vi "Unit Test Preserve wired non-serialized data (Less-Specific) True Error.vi"() -> ()   [LabVIEW 2019, in "Sports Unit Tests.lvclass"]
uses:
  Sports Unit Tests.lvclass
  <userlib>/Blue Origin/BlueSerialization/BlueSerializer/DeserializeOptions.ctl
  <userlib>/Blue Origin/BlueSerialization/BlueSerializer/DeserializeSlicingOptions.ctl
  <userlib>/Blue Origin/BlueSerialization/BlueSerializer/DeserializeMutationOptions.ctl
  <userlib>/Blue Origin/BlueSerialization/BlueSerializer/DeserializePreservationOptions.ctl
  <userlib>/Blue Origin/BlueSerialization/BlueSerializer/PreserveNonWiredDataOption.ctl
  Classes/The Waterboy/The Waterboy.lvclass
  C:/DSCE code/Serialization/blueserializationdemo/Test/Sports/Classes/Human/Human.lvclass
  C:/DSCE code/Serialization/blueserializationdemo/Test/Sports/Classes/Sports Player/Sports Player.lvclass
  C:/DSCE code/Serialization/blueserializationdemo/Test/Sports/Classes/Golf Player/Golf Player.lvclass
  C:/DSCE code/Serialization/blueserializationdemo/Test/Sports/Classes/Adam Sandler/Adam Sandler.lvclass
  Classes/Adam Sandler/Adam Sandler.lvclass
  Classes/Human/Human.lvclass/Human.ctl
  Classes/Sports Player/Sports Player.lvclass/Sports Player.ctl
  Classes/Golf Player/Golf Player.lvclass/Golf Player.ctl
  Classes/Adam Sandler/Adam Sandler.lvclass/Adam Sandler.ctl
  Classes/Human/Write Age (years).vi
  Classes/Human/Write alive_.vi
  Classes/Human/Write Height (ft).vi
  Classes/Human/Write Name.vi
  Classes/Sports Player/Write Earnings (dollars).vi
  Classes/Sports Player/Write Professional_.vi
  Classes/Sports Player/Write Sponsor.vi
  Classes/Golf Player/Write # holes in one.vi
  Classes/Golf Player/Write League.vi
  Classes/Golf Player/Write longest drive (ft).vi
  Classes/Adam Sandler/Write Movie Name.vi
  Classes/Adam Sandler/Write Private number.vi
  Classes/Adam Sandler/Write Secret phrase.vi
  <vilib>/Utility/error.llb/Clear Errors.vi
  <vilib>/Utility/LVClass/Get LV Class Name.vi
  <vilib>/addons/_JKI Toolkits/Caraya/classes/Test/Define Test.vi
  <vilib>/addons/_JKI Toolkits/Caraya/classes/Assert/Assert.vi
  <vilib>/addons/_JKI Toolkits/Caraya/classes/Assert/Assert Error.vi
  <vilib>/addons/_JKI Toolkits/Caraya/classes/Assert/Assert Equal Value_Variant.vi
  <userlib>/Blue Origin/BlueSerialization/BlueSerializer/BlueSerializer.lvclass
panel:
  out "Table":string[][](table)
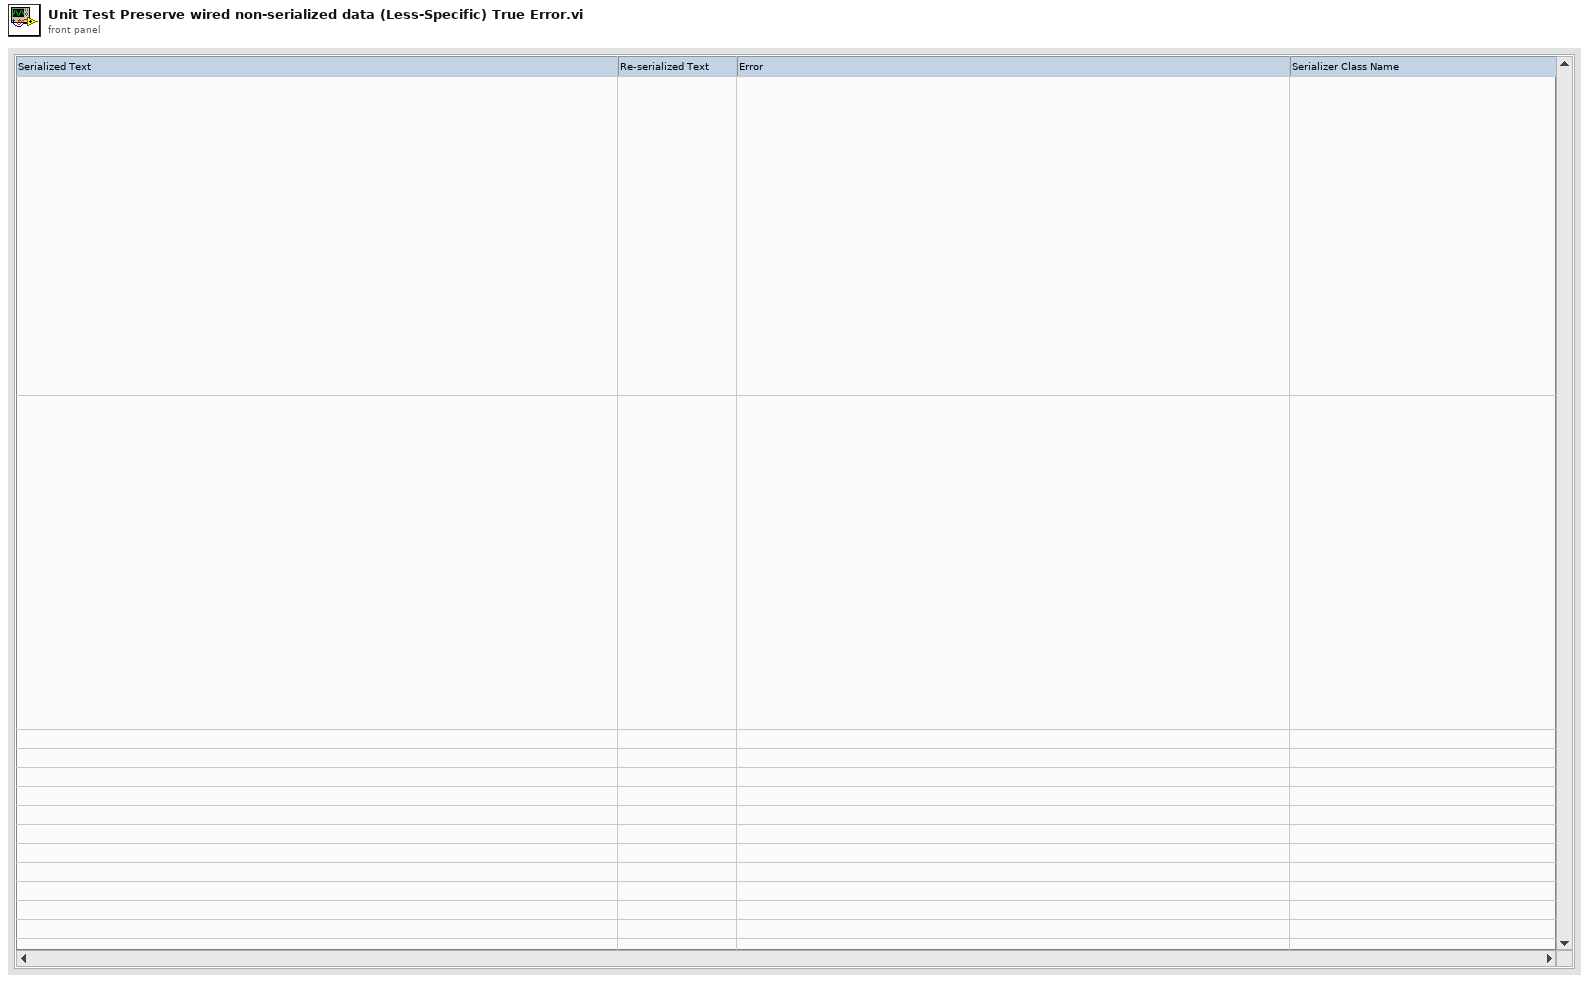
[diagram p1: front panel]
types:
  T1 = typedef "BlueSerialization.lvlib/BlueSerializer.lvclass/PreserveNonWiredDataOption.ctl" = enum16{"Don't preserve", "Preserve (error on less-specific wired types)", "Preserve (except on less-specific wired types)"}
  T2 = typedef "BlueSerialization.lvlib/BlueSerializer.lvclass/DeserializeOptions.ctl" = cluster{"deserialize non-BlueSerializable objects from hex?":bool, "expand objects on type conflict?":bool, "Slicing":T3, "Mutation Options":T4, "Preservation Options":T5}
  T3 = typedef "BlueSerialization.lvlib/BlueSerializer.lvclass/DeserializeSlicingOptions.ctl" = cluster{"slice flattened object data on error?":bool, "sliceable class names":string[]}
  T4 = typedef "BlueSerialization.lvlib/BlueSerializer.lvclass/DeserializeMutationOptions.ctl" = cluster{"error on inserted parent levels?":bool, "\terror on obsolete parent levels?":bool}
  T5 = typedef "BlueSerialization.lvlib/BlueSerializer.lvclass/DeserializePreservationOptions.ctl" = cluster{"Preserve wired serialized data?":bool, "Preserve wired non-serialized data":T1}
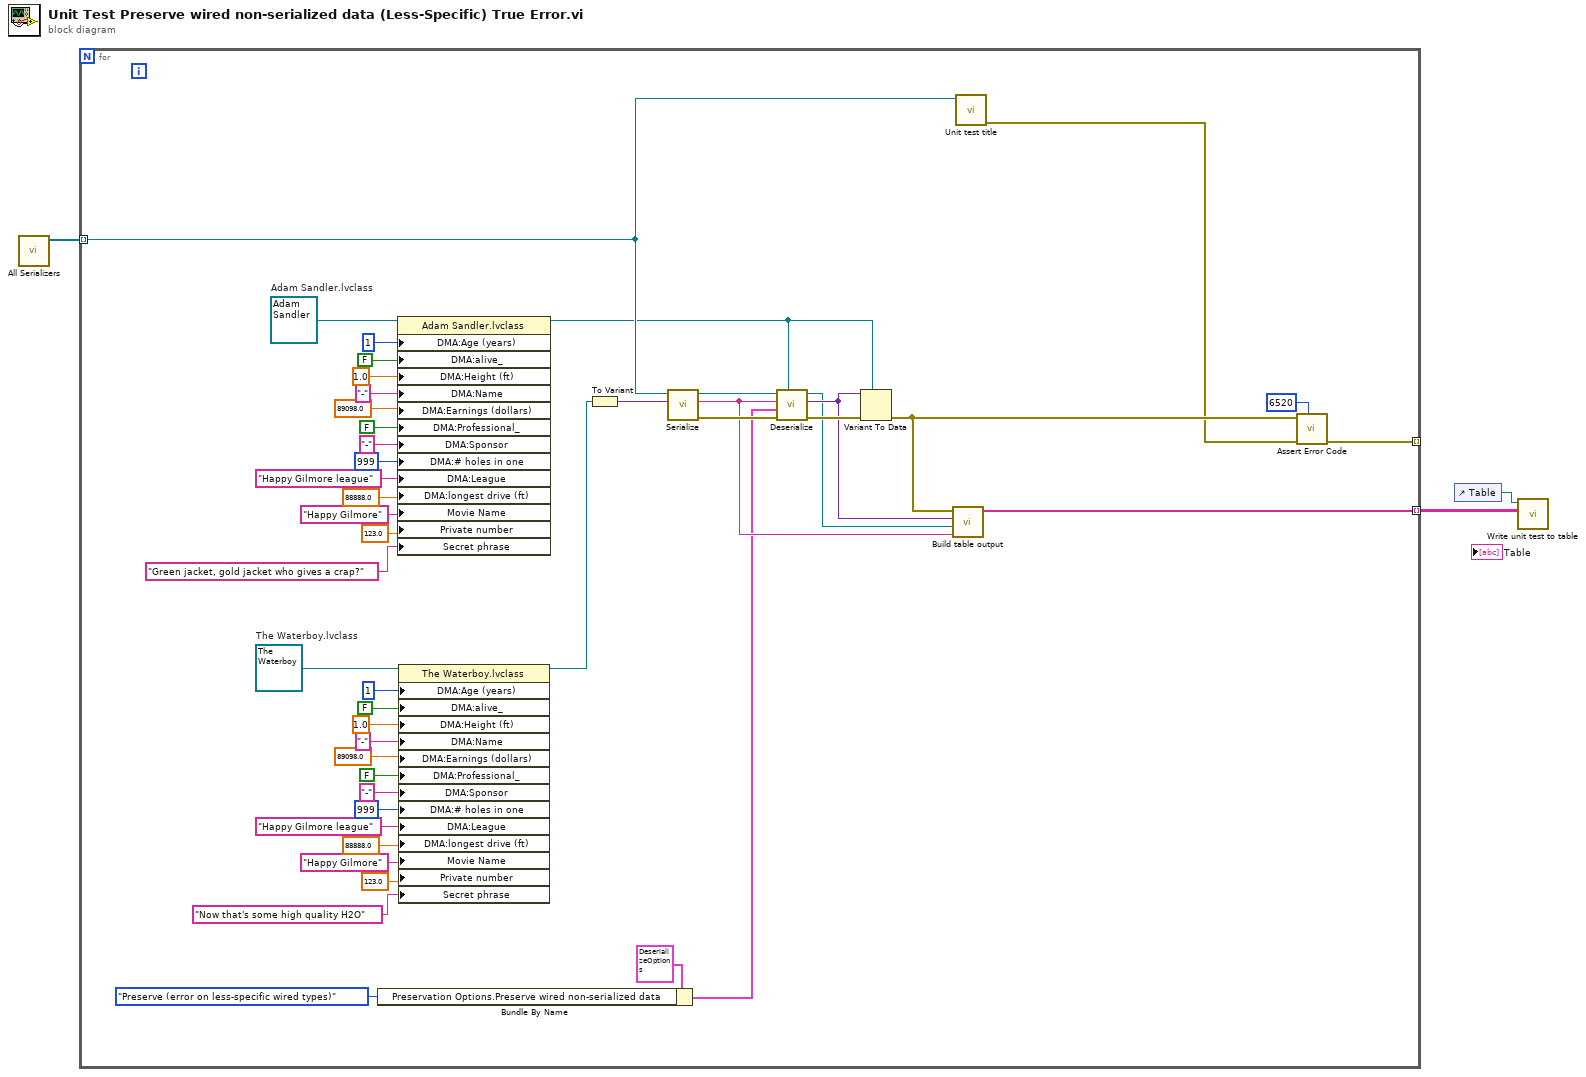
[diagram p0: block diagram]
diagram:
  n1 = call "All Serializers.vi"() -> ("All serializers"=w2:refnum<class "BlueSerializer.lvclass">[])  [unwired: 11 in]
  n2 = for {
    tunnel: w2 -> [w26] mode=indexing
    tunnel: [w5] -> _ mode=indexing
    tunnel: [w35] -> w1 mode=indexing
    w9 = refnum<class "Adam Sandler.lvclass"> refnum  # Adam Sandler.lvclass
    w10 = refnum<class "The Waterboy.lvclass"> refnum  # The Waterboy.lvclass
    n3 = Bundle By Name(cluster=T2 {"deserialize non-BlueSerializable objects from hex?"=FALSE, "expand objects on type conflict?"=FALSE, "Slicing"={"slice flattened object data on error?"=FALSE, "sliceable class names"=[]}, "Mutation Options"={"error on inserted parent levels?"=FALSE, "\terror on obsolete parent levels?"=FALSE}, "Preservation Options"={"Preserve wired serialized data?"=FALSE, "Preserve wired non-serialized data"=enum."Don't preserve"}} ("Deserialize Options"), "Preservation Options.Preserve wired non-serialized data"=PreserveNonWiredDataOption."Preserve (error on less-specific wired types)") -> (w27:T2)
    n4 = property on="Property Node" class="Adam Sandler.lvclass"(reference=w9, "DMA:Age (years)"=u16 1 ("Age (years)"), "DMA:alive_"=FALSE ("alive_"), "DMA:Height (ft)"=1.0 ("Height (ft)"), "DMA:Name"="-" ("Name"), "DMA:Earnings (dollars)"=89098.0 ("Earnings (dollars)"), "DMA:Professional_"=FALSE ("Professional_"), "DMA:Sponsor"="-" ("Sponsor"), "DMA:# holes in one"=999 ("# holes in one"), "DMA:League"="Happy Gilmore league" ("League"), "DMA:longest drive (ft)"=88888.0 ("longest drive (ft)"), "Movie Name"="Happy Gilmore", "Private number"=123.0, "Secret phrase"="Green jacket, gold jacket who gives a crap?") -> (reference out=w11:refnum<class "Adam Sandler.lvclass">)  [unwired: 1 in, 1 out]
    n5 = property on="Property Node" class="The Waterboy.lvclass"(reference=w10, "DMA:Age (years)"=u16 1 ("Age (years)"), "DMA:alive_"=FALSE ("alive_"), "DMA:Height (ft)"=1.0 ("Height (ft)"), "DMA:Name"="-" ("Name"), "DMA:Earnings (dollars)"=89098.0 ("Earnings (dollars)"), "DMA:Professional_"=FALSE ("Professional_"), "DMA:Sponsor"="-" ("Sponsor"), "DMA:# holes in one"=999 ("# holes in one"), "DMA:League"="Happy Gilmore league" ("League"), "DMA:longest drive (ft)"=88888.0 ("longest drive (ft)"), "Movie Name"="Happy Gilmore", "Private number"=123.0, "Secret phrase"="Now that's some high quality H2O") -> (reference out=w12:refnum<class "The Waterboy.lvclass">)  [unwired: 1 in, 1 out]
    n6 = To Variant(anything=w12) -> (Variant=w47:variant)
    n7 = call <userlib>:"Serialize.vi"("Anything"=w47, "BlueSerializer in"=w26) -> ("error out"=w49:errorcluster, "Serialized Text"=w36:string, "BlueSerializer out"=w48:refnum<class "BlueSerializer.lvclass">)  [unwired: 7 in]
    n8 = call <userlib>:"Deserialize.vi"("Anything"=w11, "error in (no error)"=w49, "Deserialize Options"=w27, "Serialized Text"=w36, "BlueSerializer in"=w48) -> ("error out"=w46:errorcluster, "Variant"=w38:variant, "BlueSerializer out"=w37:refnum<class "BlueSerializer.lvclass">)  [unwired: 4 in]
    n9 = Variant To Data(error in=w46, type=w11, Variant=w38) -> (error out=w7:errorcluster)  [unwired: 1 out]
    n10 = call "Build table output.vi"("serialized text"=w36, "BlueSerializer in"=w37, "deserialized variant"=w38, "variant to data error"=w7) -> ("table output"=w35:string[])  [unwired: 7 in]
    n11 = call "Unit test title.vi"("serializer"=w26) -> ("error out"=w6:errorcluster)  [unwired: 9 in, 1 out]
    n12 = call "Assert Error Code.vi"("Assert specific error code"=6520, "error in (no error)"=w6, "Error?"=w7) -> ("error out"=w5:errorcluster)  [unwired: 8 in]
  }
  n13 = control-ref of="Table"() -> (w3:refnum<vi>)
  n14 = call "Write unit test to table.vi"("Table"=w1, "Table ref in"=w3) -> ()  [unwired: 9 in, 1 out]
